vi "UDPreceiver.vi"(6 "sender's port":u16=61556, 7 "receiver's port":u16=61557, 9 "timeout ms (5000)":i32=8000, 10 "sender's IP":string="192.168.11.3", 11 "r-t":bool=TRUE) -> (0 "error":bool, 3 "data out":string)   [LabVIEW 2024]
doc: "The UDP protocol differs from TCP in that there is no error-checking with the packets of information that are sent, and thus no guarantee whatsoever that an intended recipient will actually receive a given piece of data.\n\nUDP does offer the ability to \"broadcast\" data across a network--simply specify an IP Address of all ones (255.255.255.255) to attempt to broadcast information network-wide. Keep in mind that routers and other network hardware will generally refuse to forward the broadcast beyond certain points, so the extent of the broadcast will in practice be limited."
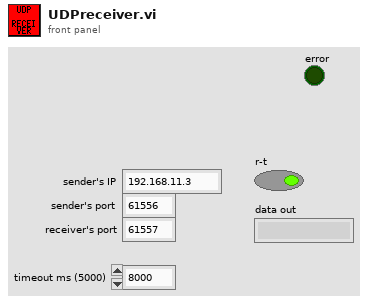
[diagram p1: front panel]
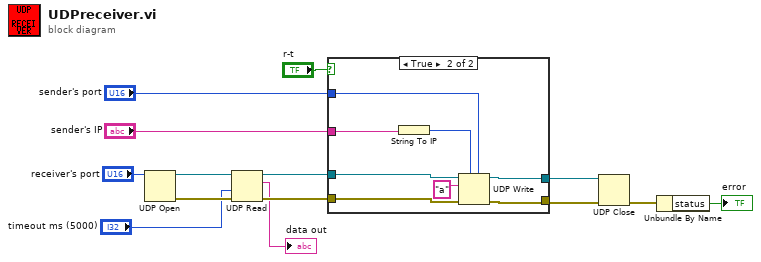
[diagram p0: block diagram]
diagram:
  n1 = UDP Open(11:"receiver's port") -> (port=w13:refnum<k16>, 0:w14:errorcluster)  [unwired: 4 in, 1 out]
  n2 = UDP Read(connection ID=w13, timeout ms (25000)="timeout ms (5000)", 8:w14) -> (data out=→"data out":string, error out=w8:errorcluster, 3:w9:refnum<k16>)  [unwired: 3 out]
  n3 = case shown="True" "r-t" {
    tunnel: [w16 w24] -> w11
    tunnel: [w15 w23] -> w10
    tunnel: w9 -> [w16 w21]
    tunnel: w8 -> [w15 w19]
    tunnel: "sender's IP" -> [_ w18]
    tunnel: "sender's port" -> [_ w17]
    frame False {
    }
    frame True {
      n4 = String To IP(1:w18) -> (0:w22:u32)
      n5 = UDP Write(address=w22, port or service name=w17, connection ID=w21, data in="a", 8:w19) -> (error out=w23:errorcluster, 3:w24:refnum<k16>)  [unwired: 1 in]
    }
  }
  n6 = UDP Close(connection ID=w11, 8:w10) -> (error out=w2:errorcluster)  [unwired: 1 out]
  n7 = Unbundle By Name(w2) -> ("status"=→"error":bool)
